vi "FVI_Manette_Process.vi"(0 "Axe L X":dbl, 1 "Axe R X":dbl, 3 "Axe L Y":dbl, 7 "Ltrigger":dbl, 9 "Rtrigger":dbl, 12 "POV":dbl, 14 "Axe R Y":dbl) -> (4 "SwerveDrive":T1)   [LabVIEW 2018]
uses:
  SwerveDrive.ctl
panel:
  out "ARD":dbl(knob) scale=-180.0..180.0
  out "ARG":dbl(knob) scale=-180.0..180.0
  out "AVD":dbl(knob) scale=-180.0..180.0
  out "AVG":dbl(knob) scale=-180.0..180.0
  out "error out":errorcluster
  in  "error in (no error)":errorcluster
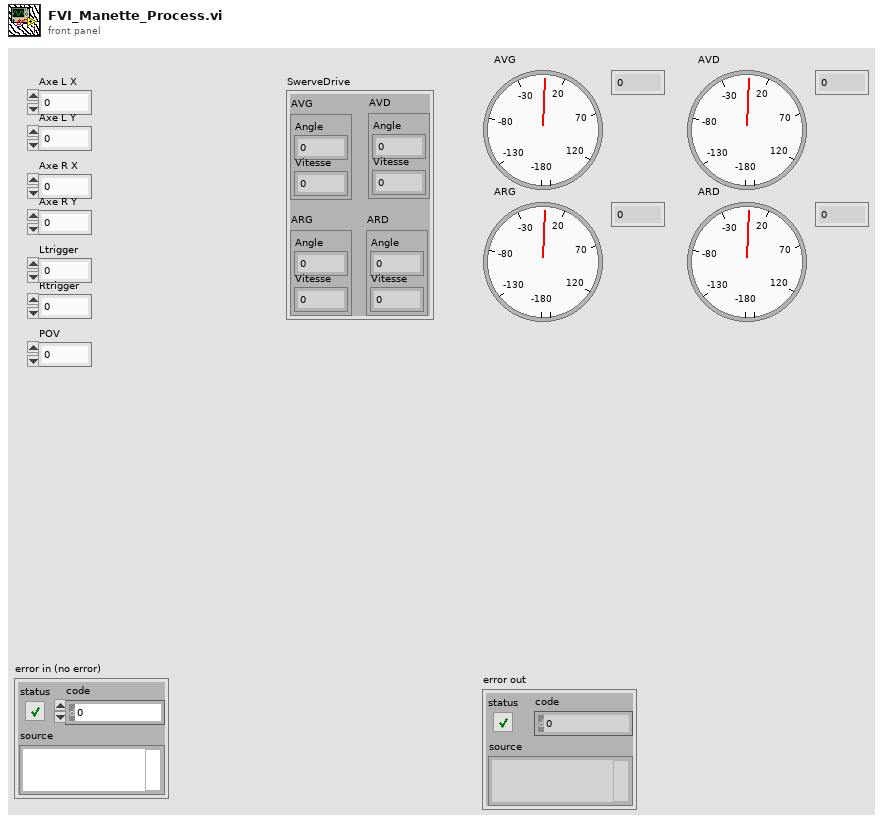
[diagram p1: front panel]
types:
  T1 = typedef "SwerveDrive.ctl" = cluster{"AVD":cluster{"Angle":dbl, "Vitesse":dbl}, "AVG":cluster{"Angle":dbl, "Vitesse":dbl}, "ARG":cluster{"Angle":dbl, "Vitesse":dbl}, "ARD":cluster{"Angle":dbl, "Vitesse":dbl}}
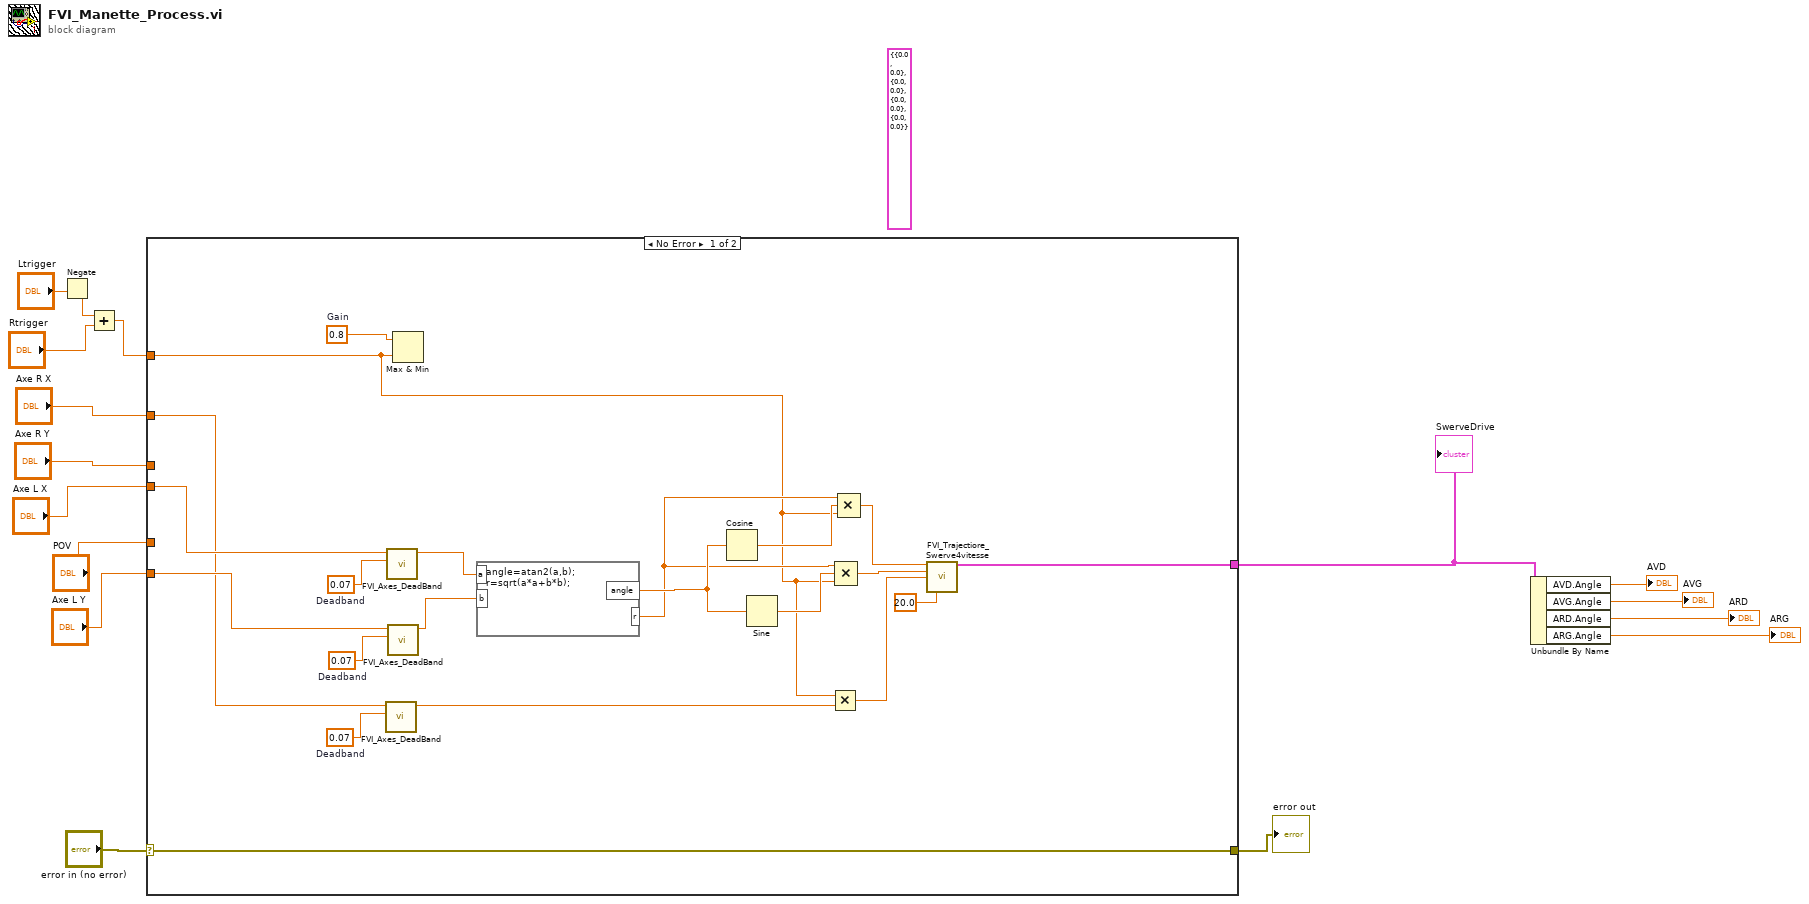
[diagram p0: block diagram]
diagram:
  (unwired) T1 {"AVD"={"Angle"=0.0, "Vitesse"=0.0}, "AVG"={"Angle"=0.0, "Vitesse"=0.0}, "ARG"={"Angle"=0.0, "Vitesse"=0.0}, "ARD"={"Angle"=0.0, "Vitesse"=0.0}} ("SwerveDrive")
  n1 = Negate(x="Ltrigger") -> (-x=w10:dbl)
  n2 = Add(x=w10, y="Rtrigger") -> (x+y=w8:dbl)
  n3 = case shown="No Error" "error in (no error)" {
    selector: "error in (no error)" -> [w37 w38]
    tunnel: "Axe L X" -> [w36 _]
    tunnel: "Axe L Y" -> [w35 _]
    tunnel: [w37 w38] -> w14
    tunnel: w8 -> [w19 _]
    tunnel: "POV" -> [_ _]
    tunnel: "Axe R X" -> [w34 _]
    tunnel: "Axe R Y" -> [_ _]
    tunnel: [w33 _] -> w5
    frame No Error {
      w27 = 0.07  # Deadband
      w29 = 0.07  # Deadband
      w31 = 0.07  # Deadband
      w32 = 0.8  # Gain
      n4 = call "FVI_Axes_DeadBand.vi"("deadband Value"=w27, "X axis in"=w34) -> ("X axis out"=w18:dbl)  [unwired: 8 in, 1 out]
      n5 = call "FVI_Axes_DeadBand.vi"("deadband Value"=w31, "X axis in"=w36) -> ("X axis out"=w30:dbl)  [unwired: 8 in, 1 out]
      n6 = call "FVI_Axes_DeadBand.vi"("deadband Value"=w29, "X axis in"=w35) -> ("X axis out"=w28:dbl)  [unwired: 8 in, 1 out]
      n7 = Max & Min(x=w32, y=w19) -> ()  [unwired: 2 out]
      n8 = formula code="angle=atan2(a,b);\nr=sqrt(a*a+b*b);"("a"=w30, "b"=w28) -> ("angle"=w25:dbl, "r"=w22:dbl)
      n9 = Cosine(x=w25) -> (cos(x)=w24:dbl)
      n10 = Sine(x=w25) -> (sin(x)=w21:dbl)
      n11 = Multiply(x=w19, y=w18) -> (x*y=w17:dbl)
      n12 = Compound Arithmetic op=MULTIPLY(w22, w21, w19) -> (w20:dbl)
      n13 = Compound Arithmetic op=MULTIPLY(w22, w24, w19) -> (w23:dbl)
      n14 = call "FVI_Trajectiore_Swerve4vitesse.vi"("Vx"=w23, "Vy"=w20, "Omega"=w17, "Distance"=20.0) -> ("SwerveDrive"=w33:T1)  [unwired: 11 in]
    }
    frame Error {
    }
  }
  "error out" <- w14
  "SwerveDrive" <- w5
  n15 = Unbundle By Name(w5) -> ("AVD.Angle"=→"AVD":dbl, "AVG.Angle"=→"AVG":dbl, "ARD.Angle"=→"ARD":dbl, "ARG.Angle"=→"ARG":dbl)
